vi "Dashboard Main.vi"() -> ()   [LabVIEW 2018]
uses:
  <vilib>/Utility/miscctls.llb/LVRowAndColumnTypeDef.ctl
  <vilib>/event_ctls.llb/eventvkey.ctl
  <vilib>/Rock Robotics/Network Tables/NT Read Numeric Array.vi
  <vilib>/Rock Robotics/WPI/Dashboard/WPI_DashboardLogging Global.vi
panel:
  in  "Camera Settings Right":T1={"Frame Rate"=30, "Compression"=30, "Size"=1, "DB Camera Config"=FALSE} {"Frame Rate" scale=1.0..30.0; "Compression" scale=100.0..-1.0; "Size" items=["640x480", "320x240", "160x120"]}
  in  "Camera Name Right":string(combo)="No Camera Selection"
  out "Camera Perf":string
  in  "Camera Settings":T1={"Frame Rate"=30, "Compression"=30, "Size"=1, "DB Camera Config"=FALSE} {"Frame Rate" scale=1.0..30.0; "Compression" scale=100.0..-1.0; "Size" items=["640x480", "320x240", "160x120"]}
  in  "TCP":refnum<k5>
  in  "Rec Mode":enum32{"Stop", "Record", "Playback"}(radio)
  out "Robot IP":string
  out "Image Message":string="Timeout in Camera Communications"
  in  "Dashboard Tab":T2(tab)=enum."Custom"
  in  "Select Auto":string(combo)="Select Autonomous ..."
  out "NT Connection":bool
  out "MotorChart R":cluster{"Numeric":dbl, "Numeric":dbl}(graph)
  out "MotorChart L":cluster{"Numeric":dbl, "Numeric":dbl}(graph)
  out "MotorSliders R":cluster{"MotorSlide1":dbl, "MotorSlide2":dbl} {"MotorSlide2" scale=-1.0..1.0 scale format="%#_2e"; "MotorSlide1" scale=-1.0..1.0 scale format="%#_2e"}
  out "MotorSliders L":cluster{"MotorSlide1":dbl, "MotorSlide2":dbl} {"MotorSlide2" scale=-1.0..1.0 scale format="%#_2e"; "MotorSlide1" scale=-1.0..1.0 scale format="%#_2e"}
  out "Gyro":dbl(knob) scale=0.0..360.0
  out "JS1 Z":dbl(slide) scale=-1.0..1.0 scale format="%#_2e"
  out "JS1 Graph":cluster{"X":dbl, "Y":dbl}[](graph)
  out "JS1 Buttons":T3
  out "JS2 Z":dbl(slide) scale=-1.0..1.0 scale format="%#_2e"
  out "JS2 Graph":cluster{"X":dbl, "Y":dbl}[](graph)
  out "JS2 Buttons":T3
  out "Mode":T4(ring)=enum."Auto Disabled"
  out "Right Camera Perf":cluster{"Bandwidth (Mbps)":dbl, "FPS":dbl}
  out "Camera Image Right":T5(plugin-control)
  in  "DB/String 9":string
  in  "DB/String 8":string
  in  "DB/String 7":string
  in  "DB/String 6":string
  in  "DB/String 5":string
  in  "DB/String 4":string
  in  "DB/String 3":string
  in  "DB/String 2":string
  in  "DB/String 1":string
  in  "DB/String 0":string
  in  "DB/Slider 0":dbl(slide) scale=0.0..5.0
  in  "DB/Slider 1":dbl(slide) scale=0.0..5.0
  in  "DB/Slider 2":dbl(slide) scale=0.0..5.0
  in  "DB/Slider 3":dbl(slide) scale=0.0..5.0
  out "DB/LED 3":bool
  out "DB/LED 2":bool
  out "DB/LED 1":bool
  out "DB/LED 0":bool
  in  "DB/Button 3":bool
  in  "DB/Button 2":bool
  in  "DB/Button 1":bool
  in  "DB/Button 0":bool caption="New Name"
  in  "Drift":dbl min=-5.0 max=5.0 step=0.1 format="%#_2g"
  in  "Rabbit":dbl=10.0 min=7.0 max=10.0 step=0.5
  in  "Speed":dbl=7.500000000000009 min=6.0 max=10.0 step=0.1 format="%#_2g"
  in  "Turtle":dbl=6.5 min=5.0 max=10.0 step=0.5 format="%#.1g"
  in  "Lift Speed":dbl=7.5 min=1.0 max=10.0 step=0.1
  in  "Tilt Speed":dbl=7.5 min=1.0 max=10.0 step=0.1
  in  "Kick Delay":dbl=0.05 min=0.05 max=1.0 step=0.05
  in  "Test Slider":dbl(slide) scale=0.0..100.0 scale format="%#_3g"
  in  "On/Off":bool caption="Solenoid"
  in  "Test Name":u16(ring) items=["Select the test to run..."]
  in  "Test Tree":string(tree)
  in  "Motor":cluster{"Value":dbl, "Enable":bool} {"Value" scale=-1.0..1.0 scale format="%#_3g"}
  out "Progress":T6 {"Test Progress" scale=0.0..100.0}
  in  "Rev/Fwd":cluster{"Forward":bool, "Reverse":bool}
  in  "Test Ring":u16(ring) items=["Monochrome", "Color"]
  out "Cmd Status":string
  in  "Execute Command":bool
  in  "Command Params":string[][](table)
  in  "Command Selection":i32(listbox)
  in  "CheckList":i32(listbox)
  out "Tree":string(tree)
  out "Camera Image":T5(plugin-control)
  out "Background":bool
  in  "Camera Name":string(combo)="No Camera Selection"
  # "HW"
  # "HW"
  # "Joysticks"
  # "Drive Motors"
  # "Front"
  # "Right"
  # "Left"
  # "Back"
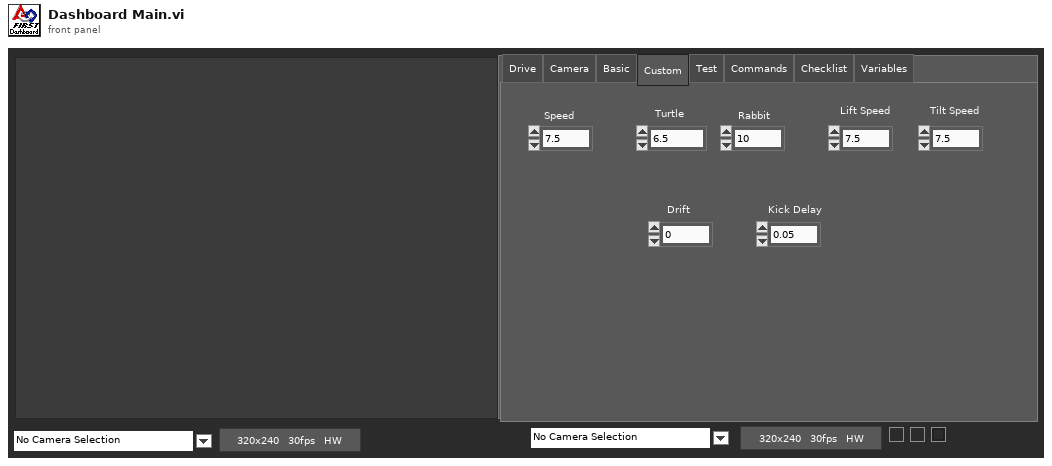
[diagram p1: front panel]
types:
  T1 = cluster{"Frame Rate":i32, "Compression":i32, "Size":u16, "DB Camera Config":bool}
  T2 = enum32{"Drive", "Camera", "Basic", "Custom", "Test", "Commands", "Checklist", "Variables"}
  T3 = cluster{bool, bool, bool, bool, bool, bool, bool, bool, bool, bool, bool, bool}
  T4 = enum8{"Tele-Op Disabled", "Tele-Op Enabled", "Auto Disabled", "Auto Enabled", "Test Disabled", "Test Enabled", "Disconnected", "No Code", "E-Stop"}
  T5 = typedef "IMAQ Image.ctl" = refnum<image>
  T6 = cluster{"Test Progress":u8, "Test Progress Text":string}
  T7 = cluster{"Save Path":path, "Interval (s)":dbl, "Keep":i32}
  T8 = typedef "Image Type" = u32
  T9 = cluster{"IDs":cluster{"RPC field ID":u16, "Unique ID":u16}, "String":string}
  T10 = cluster{"Error Strings":string, "Disable Counts":cluster{u16, u16}, "Rail Faults":cluster{u16, u16, u16}, "Robot IP":string, "DB Mode":u8, "Event Info":cluster{"Name":string, "Type":u8, "Number":u16, "Replay":u8}}
  T11 = cluster{"Storage":cluster{"Disk Free":u64, "RAM Block":u32, "RAM free":u32}, "CPU Utilization":cluster{"CPU % ISR":sgl, "CPU % Time Crit":sgl, "CPU % Timed Str":sgl, "CPU % High":sgl, "CPU % Above":sgl, "CPU % Normal":sgl, "CPU % Low":sgl}, "CAN":cluster{"% Bus Utilization":sgl, "Bus Off Cnt":u32, "TX_FIFO Full Cnt":u32, "Receive Error Cnt":u8, "Transmit Error Cnt":u8}, "HID":cluster{"HID Outputs":u32, "Rumble Low":u16, "Rumble High":u16}[]}
  T12 = cluster{"Status bits":cluster{"Test Mode":bool, "Autonomous":bool, "Enabled":bool, "Code Start":bool, "Brownout":bool, "Reserved 2":bool, "Reserved 3":bool, "E-Stop":bool}, "Code Trace":cluster{"Disabled":bool, "TeleOp":bool, "Auto":bool, "Test":bool}, "Controller Type":enum16{"unknown", "cRIO", "roboRio"}, "Code?":enum16{"unknown", "noCode", "code"}, "Battery V":dbl}
  T13 = cluster{"Control Bits":cluster{"TestMode":bool, "Autonomous":bool, "Enabled":bool, "FMS Present":bool, bool, bool, bool, "E-Stop":bool}, "Team Station ":u8, "Countdown":sgl, "Joystick Values":cluster{"Axes":dbl[], "Buttons":bool[], "POVs":i16[]}[]}
  T14 = cluster{"Axes":dbl[], "Buttons":bool[], "POVs":i16[]}[]
  T15 = cluster{"Axes":dbl[], "Buttons":bool[], "POVs":i16[]}
  T16 = cluster{"Buttons[0]":bool, "Buttons[1]":bool, "Buttons[2]":bool, "Buttons[3]":bool, "Buttons[4]":bool, "Buttons[5]":bool, "Buttons[6]":bool, "Buttons[7]":bool, "Buttons[8]":bool, "Buttons[9]":bool, "Buttons[10]":bool, "Buttons[11]":bool}
  T17 = cluster{"Camera Image":refnum<vi>, "Dashboard Tab":refnum<vi>, "Background":refnum<vi>, "Rec Mode":refnum<vi>, "Test Slider":refnum<vi>, "On/Off ":refnum<vi>, "Test Ring":refnum<vi>, "Rev/Fwd":refnum<vi>, "Test Name":refnum<vi>, "Motor":refnum<vi>, "Progress":refnum<vi>, "CheckList":refnum<vi>, "Tree":refnum<vi>, "Test Tree":refnum<vi>, "Command Params":refnum<vi>, "Command Selection":refnum<vi>, "Execute Command":refnum<vi>, "Cmd Status":refnum<vi>, "Camera Settings":refnum<vi>, "Camera Name":refnum<vi>, "Camera Perf":refnum<vi>, "Camera Settings Right":refnum<vi>, "Camera Name Right":refnum<vi>, "Camera Image Right":refnum<vi>}
  T18 = cluster{"Global Rectangle":i32[], "Contours":cluster{"Contour Type":u32, "ROI Type":u32, "Points":i32[]}[]}
  T19 = cluster{"Camera Name Right":string, string, "Saved DB Images Info":cluster{"Save Path":path, "Interval (s)":dbl, "Keep":i32}}
  T20 = cluster{"Camera Name":string, string, "Saved DB Images Info":cluster{"Save Path":path, "Interval (s)":dbl, "Keep":i32}}
  T21 = cluster{"Operation":enum16{"Update", "Clear"}, "Color Box":u32}[]
  T22 = typedef "eventvkey.ctl" = enum16{"ASCII", "Enter", "Return", "Shift", "Ctrl", "Alt", "Cmd", "Opt", "Caps", "NumLock", "Clear", "Break", "Up", "Down", "Left", "Right", "Insert", "Delete", "Home", "End", "PageUp", "PageDown", "Escape", "Help", "Pause", "ScrollLock", "F1", "F2", "F3", "F4", "F5", "F6", "F7", "F8", "F9", "F10", "F11", "F12", "F13", "F14", "F15", "F16", "F17", "F18", "F19", "F20", "F21", "F22", "F23", "F24", "Play", "VolumeUp", "VolumeDown", "Mute", "Two Byte Char"}
  T23 = cluster{"Image Size":bool, "Image Type":bool, "Pixel Value":bool, "ROI Information":bool, "Zoom Factor":bool}
  T24 = cluster{"Operation":enum16{"Update", "Clear"}, "Color Box":u32}
  T25 = typedef "LVRowAndColumnTypeDef.ctl" = cluster{"Row":i32, "Column":i32}
  T26 = cluster{"Shift":bool, "Ctrl":bool, "Alt":bool, "Cmd":bool, "Opt":bool}
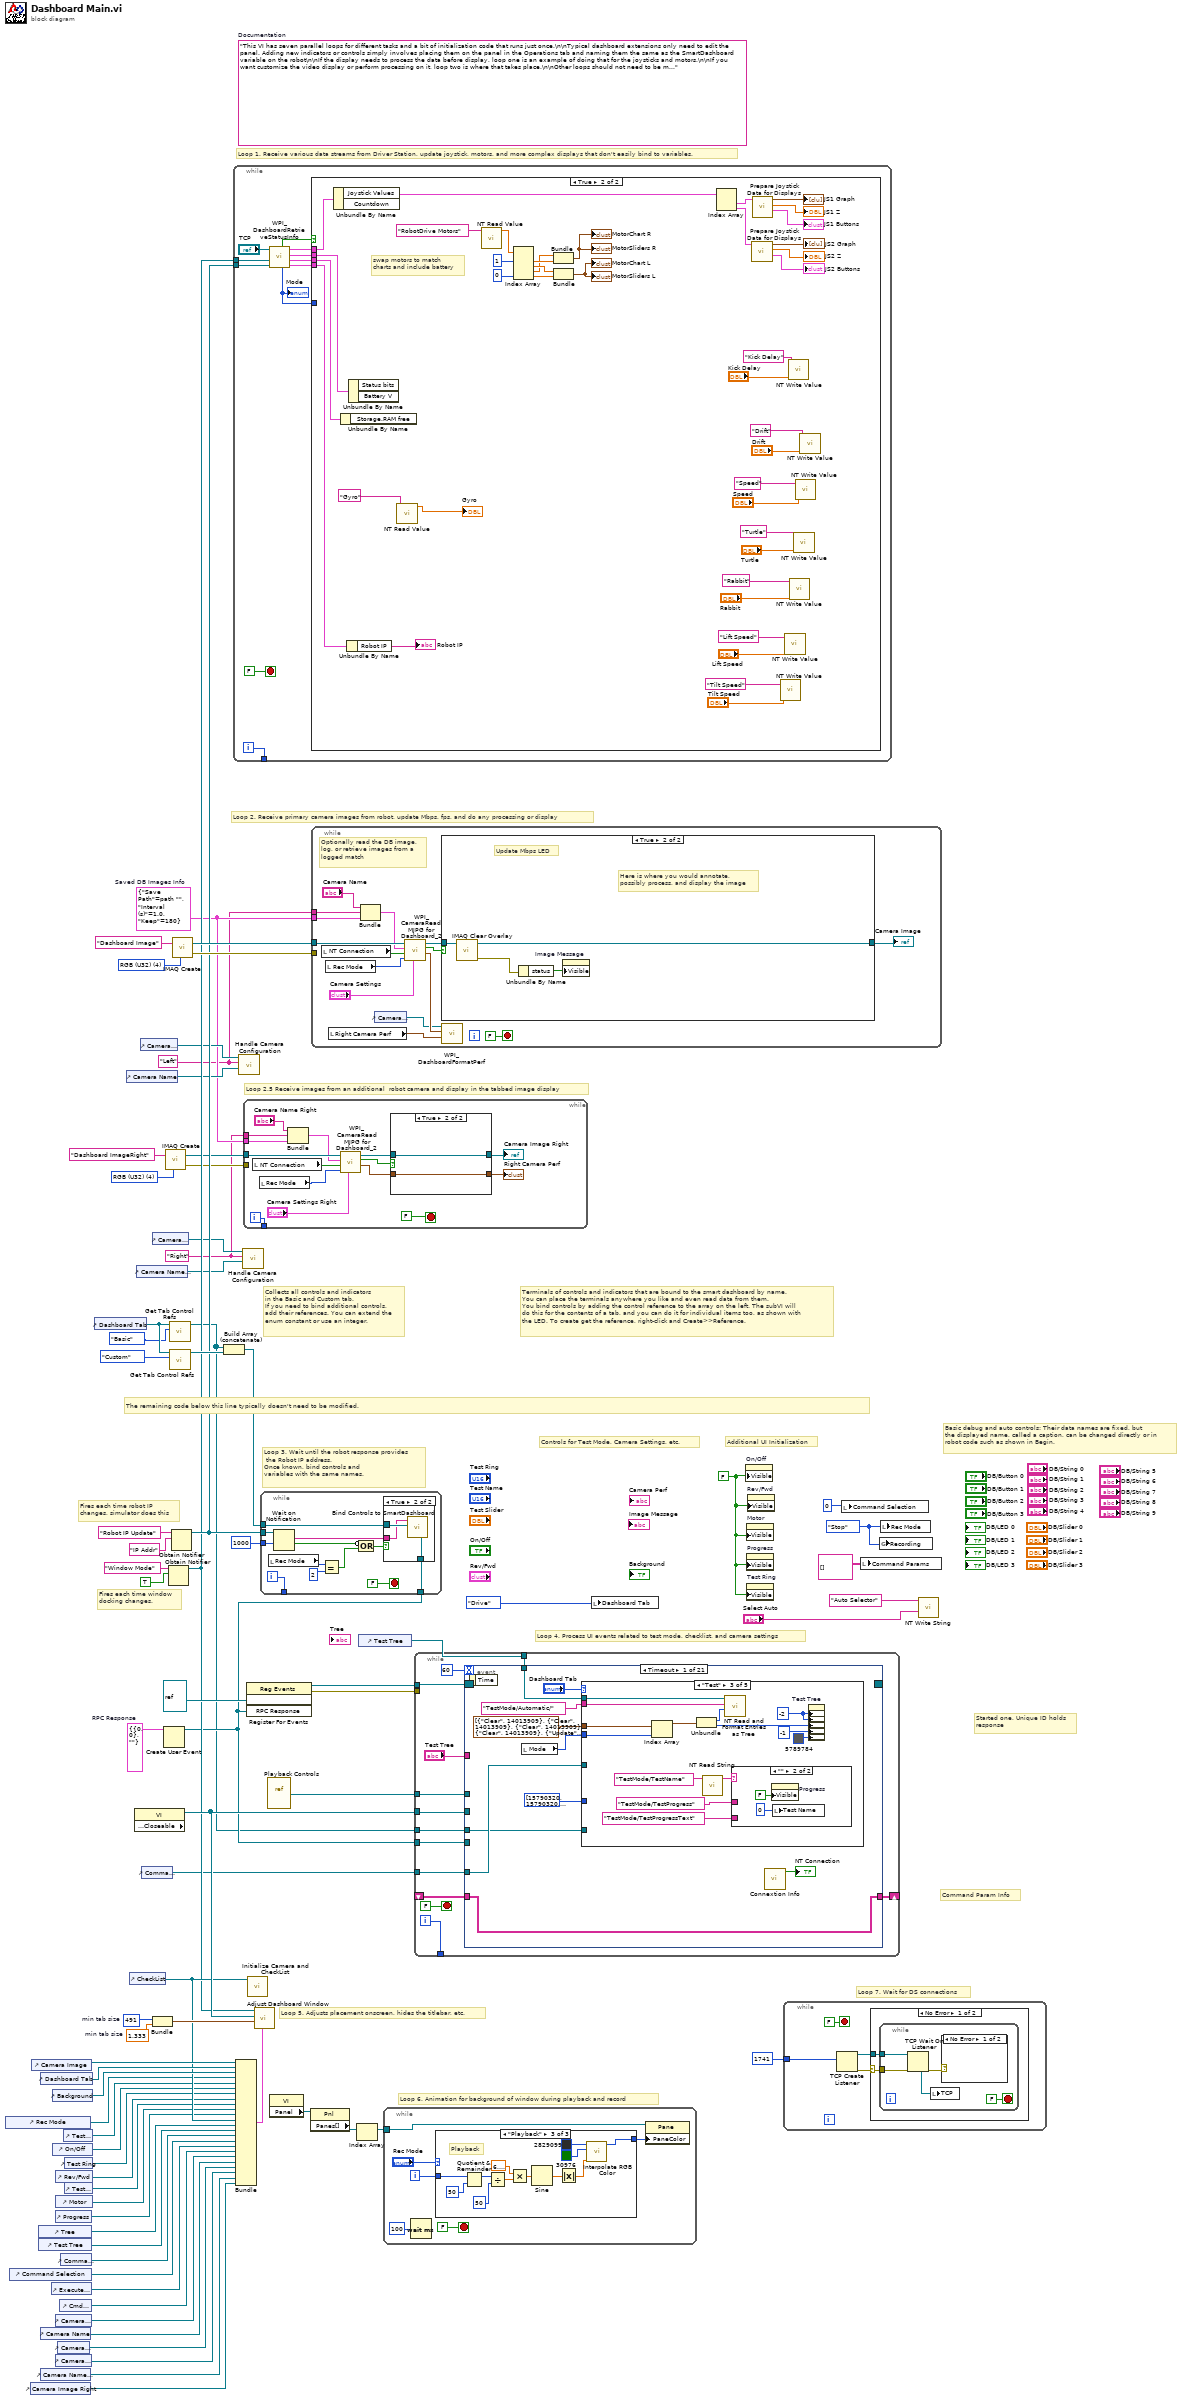
[diagram p0: block diagram]
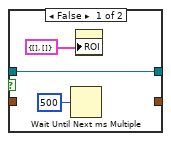
[diagram p2: hidden frame]
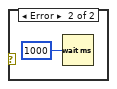
[diagram p3: hidden frame]
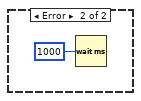
[diagram p4: hidden frame]
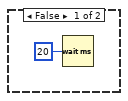
[diagram p5: hidden frame]
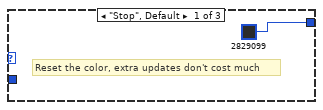
[diagram p6: hidden frame]
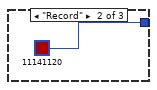
[diagram p7: hidden frame]
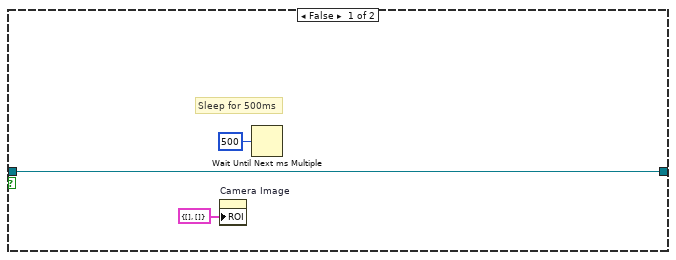
[diagram p9: hidden frame]
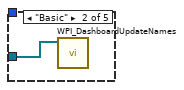
[diagram p11: hidden frame]
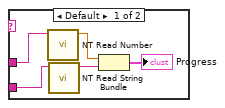
[diagram p12: hidden frame]
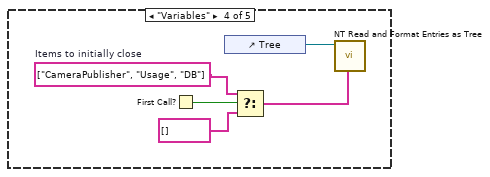
[diagram p13: hidden frame]
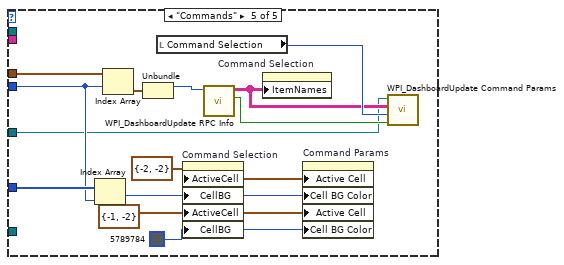
[diagram p14: hidden frame]
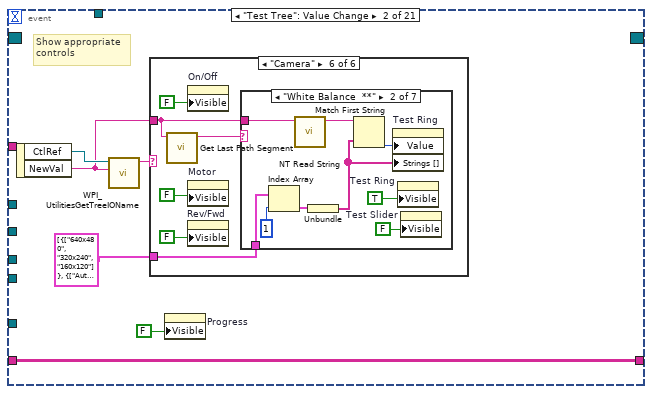
[diagram p15: hidden frame]
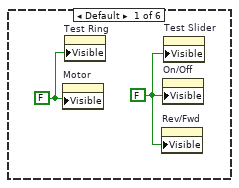
[diagram p16: hidden frame]
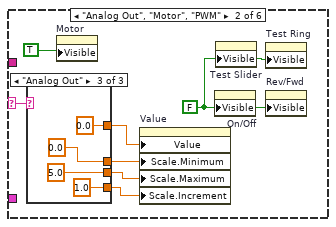
[diagram p17: hidden frame]
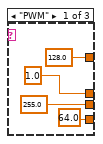
[diagram p18: hidden frame]
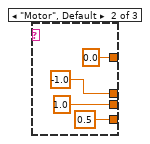
[diagram p19: hidden frame]
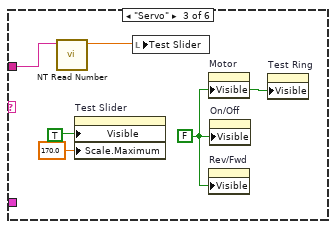
[diagram p20: hidden frame]
diagram:
  w3 = T7 {"Save Path"=path "", "Interval (s)"=1.0, "Keep"=180}  # Saved DB Images Info
  w2 = "Right"
  w1 = "Left"
  w13 = T8 4 items=["Grayscale (U8)", "Grayscale (I16)", "Grayscale (SGL)", "Complex (CSG)", "RGB (U32)", "HSL (U32)", "RGB (U64)"] ("Image Type")
  w29 = T9 {"IDs"={"RPC field ID"=0, "Unique ID"=0}, "String"=""}  # RPC Response
  w52 = 491  # min tab size
  w51 = 1.333  # min tab size
  w59 = enum32{"Stop", "Record", "Playback"}."Stop" ("Rec Mode")
  w36 = FALSE ("Visible")
  (unwired) "This VI has seven parallel loops for different tasks and a bit of initialization code that runs just once.\n\nTypical dashboard extensions only need to edit the panel. Adding new indicators or controls simply involves placing them on the panel in the Operations tab and naming them the same as the SmartDashboard variable on the robot\n\nIf the display needs to process the data before display, loop one is an example of doing that for the joysticks and motors.\n\nIf you want customize the video display or perform processing on it, loop two is where that takes place.\n\nOther loops should not need to be modified. They are pretty standard, and document the task they perform."  # Documentation
  w76 = T8 4 items=["Grayscale (U8)", "Grayscale (I16)", "Grayscale (SGL)", "Complex (CSG)", "RGB (U32)", "HSL (U32)", "RGB (U64)"] ("Image Type")
  # "Loop 2.5 Receive images from an additional  robot camera and display in the tabbed image display"
  # "Command Param Info"
  # "Started one, Unique ID holds\nresponse"
  # "Loop 7. Wait for DS connections"
  # "Basic debug and auto controls: Their data names are fixed, but\nthe displayed name, called a caption, can be changed directly or in\nrobot code such as shown in Begin."
  # "Controls for Test Mode, Camera Settings, etc."
  # "Additional UI Initialization"
  # "Loop 6. Animation for background of window during playback and record"
  # "Fires each time robot IP\nchanges, simulator does this"
  # "Fires each time window\ndocking changes."
  # "Collects all controls and indicators\nin the Basic and Custom tab.\nIf you need to bind additional controls,\nadd their references. You can extend the\nenum constant or use an integer."
  # "The remaining code below this line typically doesn't need to be modified."
  # "Loop 4. Process UI events related to test mode, checklist, and camera settings"
  # "Terminals of controls and indicators that are bound to the smart dashboard by name.\nYou can place the terminals anywhere you like and even read data from them.\nYou bind controls by adding the control reference to the array on the left. The subVI will\ndo this for the contents of a tab, and you can do it for individual items too, as shown with\nthe LED. To create get the reference, right-click and Create>>Reference."
  # "Loop 3. Wait until the robot response provides\n the Robot IP address.\nOnce known, bind controls and\nvariables with the same names."
  # "Loop 5. Adjusts placement onscreen, hides the titlebar, etc."
  # "Loop 1. Receive various data streams from Driver Station, update joystick, motors, and more complex displays that don't easily bind to variables."
  # "Loop 2. Receive primary camera images from robot, update Mbps, fps, and do any processing or display"
  n1 = control-ref of="Rec Mode"() -> (w42:refnum<vi>)
  n2 = control-ref of="Command Selection"() -> (w28:refnum<vi>)
  n3 = control-ref of="Camera Image Right"() -> (w6:refnum<vi>)
  n4 = control-ref of="Camera Image"() -> (w54:refnum<vi>)
  n5 = control-ref of="Tree"() -> (w46:refnum<vi>)
  n6 = control-ref of="Test Tree"() -> (w45:refnum<vi>)
  n7 = control-ref of="Dashboard Tab"() -> (w53:refnum<vi>)
  n8 = control-ref of="Camera Name"() -> (w19:refnum<vi>)
  n9 = control-ref of="Camera Name Right"() -> (w7:refnum<vi>)
  n10 = control-ref of="Execute Command"() -> (w30:refnum<vi>)
  n11 = control-ref of="Background"() -> (w49:refnum<vi>)
  n12 = control-ref of="On/Off"() -> (w40:refnum<vi>)
  n13 = control-ref of="Progress"() -> (w37:refnum<vi>)
  n14 = control-ref of="Camera Settings"() -> (w20:refnum<vi>)
  n15 = control-ref of="Camera Settings Right"() -> (w8:refnum<vi>)
  n16 = control-ref of="Rev/Fwd"() -> (w38:refnum<vi>)
  n17 = control-ref of="Motor"() -> (w43:refnum<vi>)
  n18 = control-ref of="Camera Perf"() -> (w18:refnum<vi>)
  n19 = control-ref of="Cmd Status"() -> (w24:refnum<vi>)
  n20 = control-ref of="Command Params"() -> (w31:refnum<vi>)
  n21 = control-ref of="Test Slider"() -> (w41:refnum<vi>)
  n22 = control-ref of="Test Ring"() -> (w39:refnum<vi>)
  n23 = control-ref of="Test Name"() -> (w44:refnum<vi>)
  n24 = control-ref of="Dashboard Tab"() -> (w57:refnum<vi>)
  n25 = control-ref of="Camera Name"() -> (w21:refnum<vi>)
  n26 = control-ref of="CheckList"() -> (w47:refnum<vi>)
  n27 = property class="VI" props=["Front Panel.Closeable"]() -> (reference out=w58:refnum<vi>)  [unwired: 2 in, 2 out]
  n28 = control-ref of="Camera Name Right"() -> (w9:refnum<vi>)
  n29 = control-ref of="Camera Settings"() -> (w22:refnum<vi>)
  n30 = control-ref of="Command Params"() -> (w23:refnum<vi>)
  n31 = control-ref of="Camera Settings Right"() -> (w10:refnum<vi>)
  n32 = Bundle("min tab size"=w52, "min tab size"=w51) -> (w50:cluster{"min tab size":i32, "min tab size":dbl})  [unwired: 1 in]
  n33 = Create User Event(user event datatype=w29) -> (user event=w25:refnum<user-event>)  [unwired: 1 in, 1 out]
  n34 = call "IMAQ Create"("Image Name"="Dashboard ImageRight", "Image Type"=w13) -> ("New Image"=w12:T5, "error out"=w11:errorcluster)  [unwired: 2 in, 1 out]
  n35 = Obtain Notifier(name (unnamed)="Window Mode", notification data type=TRUE) -> (notifier out=w34:refnum<notifier>)  [unwired: 2 in, 2 out]
  n36 = call <vilib>:"Get Tab Control Refs.vi"("Page Index"=T2."Basic" ("Dashboard Tab"), "TabControl in"=w57) -> ("ControlsOnPage"=w17:refnum<vi>[])  [unwired: 9 in]
  n37 = call <vilib>:"Get Tab Control Refs.vi"("Page Index"=T2."Custom" ("Dashboard Tab"), "TabControl in"=w57) -> ("ControlsOnPage"=w56:refnum<vi>[])  [unwired: 9 in]
  n38 = Obtain Notifier(name (unnamed)="Robot IP Update", notification data type="IP Addr" ("name (unnamed)")) -> (notifier out=w35:refnum<notifier>)  [unwired: 2 in, 2 out]
  n39 = call "IMAQ Create"("Image Name"="Dashboard Image", "Image Type"=w76) -> ("New Image"=w74:T5, "error out"=w73:errorcluster)  [unwired: 2 in, 1 out]
  n40 = Build Array (concatenate)(w17, w56) -> (w55:refnum<vi>[])
  n41 = while {
    tunnel: [w86] -> _
    tunnel: w35 -> [w80]
    tunnel: w34 -> [w77]
    i -> [w86]
    stop <- FALSE stop-if-true
    n42 = call <vilib>:"WPI_DashboardRetrieveStatusInfo.vi"("Binding Refnum"=w80, "Window Mode Notifier"=w77, "TCP Cnx"="TCP") -> ("Power and Errors"=w81:T10, "Robot Metrics"=w84:T11, "Status Info"=w85:T12, "Control Info"=w82:T13, "Robot Mode"=w79:T4, "Process?"=w83:bool)  [unwired: 3 in]
    "Mode" <- w79
    n43 = case shown="True" w83 {
      tunnel: w85 -> [_ w128]
      tunnel: w84 -> [_ w127]
      tunnel: w82 -> [_ w126]
      tunnel: w81 -> [_ w125]
      tunnel: w79 -> [_ _]
      frame False {
        n44 = Wait (ms)(milliseconds to wait=u32 20) -> ()  [unwired: 1 out]
      }
      frame True {
        # "swap motors to match\ncharts and include battery"
        n45 = Unbundle By Name(w126) -> ("Joystick Values"=w116:T14)  [unwired: 1 out]
        n46 = Unbundle By Name(w127) -> ()  [unwired: 1 out]
        n47 = Unbundle By Name(w125) -> ("Robot IP"=→"Robot IP":string)
        n48 = Unbundle By Name(w128) -> ()  [unwired: 2 out]
        n49 = call-poly <vilib>:"NT Read Value.vi"("Name"="Gyro") -> ("Numeric"=→"Gyro":dbl)  [unwired: 9 in, 1 out]
        n50 = call-poly <vilib>:"NT Read Value.vi"("Name"="RobotDrive Motors") -> ("Numeric Array"=w106:dbl[])  [unwired: 9 in, 1 out]
        n51 = Index Array(array=w106, index #1=1, index #4=0) -> (element #1=w120:dbl, element #2=w121:dbl, element #3=w119:dbl, element #4=w124:dbl)  [unwired: 2 in]
        n52 = Bundle("Numeric"=w119, "Numeric"=w120) -> (→"MotorChart R" →"MotorSliders R":cluster{"Numeric":dbl, "Numeric":dbl})  [unwired: 1 in]
        n53 = Bundle("Numeric"=w121, "Numeric"=w124) -> (→"MotorChart L" →"MotorSliders L":cluster{"Numeric":dbl, "Numeric":dbl})  [unwired: 1 in]
        n54 = Index Array(array=w116) -> (element #1=w115:T15, element #2=w111:T15)  [unwired: 2 in]
        n55 = call "Prepare Joystick Data for Displays.vi"("Joystick Values"=w111) -> ("Buttons"=→"JS2 Buttons":T16, "Z Axis"=→"JS2 Z":dbl, "Cartesian Data"=→"JS2 Graph":cluster{"X axis":dbl, "X axis":dbl}[])  [unwired: 8 in]
        n56 = call "Prepare Joystick Data for Displays.vi"("Joystick Values"=w115) -> ("Buttons"=→"JS1 Buttons":T16, "Z Axis"=→"JS1 Z":dbl, "Cartesian Data"=→"JS1 Graph":cluster{"X axis":dbl, "X axis":dbl}[])  [unwired: 8 in]
        n57 = call-poly <vilib>:"NT Write Value.vi"("Numeric"="Tilt Speed", "Name"="Tilt Speed") -> ()  [unwired: 9 in, 1 out]
        n58 = call-poly <vilib>:"NT Write Value.vi"("Numeric"="Lift Speed", "Name"="Lift Speed") -> ()  [unwired: 9 in, 1 out]
        n59 = call-poly <vilib>:"NT Write Value.vi"("Numeric"="Kick Delay", "Name"="Kick Delay") -> ()  [unwired: 9 in, 1 out]
        n60 = call-poly <vilib>:"NT Write Value.vi"("Numeric"="Rabbit", "Name"="Rabbit") -> ()  [unwired: 9 in, 1 out]
        n61 = call-poly <vilib>:"NT Write Value.vi"("Numeric"="Turtle", "Name"="Turtle") -> ()  [unwired: 9 in, 1 out]
        n62 = call-poly <vilib>:"NT Write Value.vi"("Numeric"="Speed", "Name"="Speed") -> ()  [unwired: 9 in, 1 out]
        n63 = call-poly <vilib>:"NT Write Value.vi"("Numeric"="Drift", "Name"="Drift") -> ()  [unwired: 9 in, 1 out]
      }
    }
  }
  n64 = Bundle("Camera Image"=w54, "Dashboard Tab"=w53, "Background"=w49, "Rec Mode"=w42, "Test Slider"=w41, "On/Off"=w40, "Test Ring"=w39, "Rev/Fwd"=w38, "Test Name"=w44, "Motor"=w43, "Progress"=w37, "CheckList"=w47, "Tree"=w46, "Test Tree"=w45, "Command Params"=w31, "Command Selection"=w28, "Execute Command"=w30, "Cmd Status"=w24, "Camera Settings"=w20, "Camera Name"=w19, "Camera Perf"=w18, "Camera Settings Right"=w8, "Camera Name Right"=w7, "Camera Image Right"=w6) -> (w48:T17)  [unwired: 1 in]
  n65 = call "Handle Camera Configuration.vi"("CameraNameRef"=w21, "Display Name"=w1, "ClusterRef"=w22) -> ()  [unwired: 9 in]
  n66 = call "Handle Camera Configuration.vi"("CameraNameRef"=w9, "Display Name"=w2, "ClusterRef"=w10) -> ()  [unwired: 9 in]
  n67 = while {
    tunnel: w12 -> [w143]
    tunnel: w11 -> [_]
    tunnel: [w138] -> _
    tunnel: w3 -> [w134]
    tunnel: w2 -> [w131]
    i -> [w138]
    stop <- FALSE stop-if-true
    n68 = local read "NT Connection"() -> (w135:bool)
    n69 = local read "Rec Mode"() -> (w142:enum32{"Stop", "Record", "Playback"})
    n70 = Bundle("Camera Name Right"="Camera Name Right", w131, "Saved DB Images Info"=w134) -> (w133:T19)  [unwired: 1 in]
    n71 = call <vilib>:"WPI_CameraRead MJPG for Dashboard_2.vi"("Camera Settings"="Camera Settings Right", "Rec Mode"=w142, "NT Connection"=w135, "Capture Info"=w133, "Image in"=w143) -> ("perf info"=w129:cluster{"Bandwidth (Mbps)":dbl, "fps":dbl}, "Active"=w137:bool, "Image\\ out"=w140:T5)  [unwired: 4 in]
    n72 = case shown="True" w137 {
      tunnel: w140 -> [w145 w148]
      tunnel: [w145 w148] -> w136
      tunnel: [_ w147] -> w130
      tunnel: w129 -> [_ w147]
      frame False {
        n73 = Wait Until Next ms Multiple(millisecond multiple=u32 500) -> ()  [unwired: 1 out]
        n74 = property on="Camera Image Right" class="ImageControl"("ROI"=T18 {"Global Rectangle"=[], "Contours"=[]}) -> ()  [unwired: 2 in, 2 out]
      }
      frame True {
      }
    }
    "Camera Image Right" <- w136
    "Right Camera Perf" <- w130
  }
  n75 = register-events(refnum<vi> refnum, w25) -> (reference out=w63:refnum<event-registration>, error out=w62:errorcluster)  [unwired: 2 in]
  n76 = call "Initialize Camera and CheckList.vi"("ListBox in"=w47) -> ()  [unwired: 11 in]
  n77 = call "Adjust Dashboard Window.vi"("Sizing Refnums"=w48, "Size Constraints"=w50, "VI"=w58, "WIn Mode"=w34) -> ()  [unwired: 8 in]
  n78 = while {
    tunnel: w55 -> [w160]
    tunnel: w35 -> [w158]
    tunnel: [w156] -> _
    tunnel: u32 1000 ("milliseconds to wait") -> [w155]
    tunnel: w25 -> [w149]
    i -> [w156]
    stop <- FALSE stop-if-true
    n79 = local read "Rec Mode"() -> (w151:enum32{"Stop", "Record", "Playback"})
    n80 = Wait on Notification(notifier=w158, timeout in ms (-1)=w155) -> (notification=w157:string, timed out?=w153:bool)  [unwired: 2 in, 2 out]
    n81 = Equal?(x=w151, y=u16 2 ("Rec Mode")) -> (x = y?=w152:bool)
    n82 = Compound Arithmetic op=OR(invert w153, w152) -> (w154:bool)
    n83 = case shown="True" w154 {
      tunnel: w160 -> [_ w163]
      tunnel: w157 -> [_ w162]
      tunnel: w149 -> [_ w161]
      frame False {
      }
      frame True {
        n84 = call <vilib>:"Bind Controls to SmartDashboard.vi"("RPC ref"=w161, "Bound Control Refs"=w163, "Server IP Address"=w162) -> ()  [unwired: 9 in]
      }
    }
  }
  n85 = vi-ref "Playback Controls.vi"() -> (w64:refnum<vi>)
  n86 = property class="VI"() -> ("Panel"=w66:refnum<vi>)  [unwired: 2 in, 2 out]
  n87 = property class="Pnl"(reference=w66) -> ("Panes[]"=w67:refnum<vi>[])  [unwired: 1 in, 2 out]
  n88 = while {
    tunnel: w74 -> [w177]
    tunnel: w73 -> [_]
    tunnel: w3 -> [w170]
    tunnel: w1 -> [w167]
    stop <- FALSE stop-if-true
    # "Optionally read the DB image,\nlog, or retrieve images from a\nlogged match"
    n89 = local read "NT Connection"() -> (w171:bool)
    n90 = local read "Rec Mode"() -> (w174:enum32{"Stop", "Record", "Playback"})
    n91 = local read "Right Camera Perf"() -> (w165:cluster{"Bandwidth (Mbps)":dbl, "FPS":dbl})
    n92 = Bundle("Camera Name"="Camera Name", w167, "Saved DB Images Info"=w170) -> (w169:T20)  [unwired: 1 in]
    n93 = control-ref of="Camera Perf"() -> (w164:refnum<vi>)
    n94 = call <vilib>:"WPI_CameraRead MJPG for Dashboard_2.vi"("Camera Settings"="Camera Settings", "Rec Mode"=w174, "NT Connection"=w171, "Capture Info"=w169, "Image in"=w177) -> ("perf info"=w166:cluster{"Bandwidth (Mbps)":dbl, "fps":dbl}, "Active"=w175:bool, "Image\\ out"=w176:T5)  [unwired: 4 in]
    n95 = case shown="True" w175 {
      tunnel: w176 -> [w180 w183]
      tunnel: [w180 w182] -> w172
      frame False {
        # "Sleep for 500ms"
        n96 = property on="Camera Image" class="ImageControl"("ROI"=T18 {"Global Rectangle"=[], "Contours"=[]}) -> ()  [unwired: 2 in, 2 out]
        n97 = Wait Until Next ms Multiple(millisecond multiple=u32 500) -> ()  [unwired: 1 out]
      }
      frame True {
        # "Here is where you would annotate,\npossibly process, and display the image"
        # "Update Mbps LED"
        n98 = call "IMAQ Clear Overlay"("Image"=w183) -> ("error out"=w184:errorcluster, "Image Out"=w182:T5)  [unwired: 2 in, 7 out]
        n99 = Unbundle By Name(w184) -> ("status"=w185:bool)
        n100 = property on="Image Message" class="Str"("Visible"=w185) -> ()  [unwired: 2 in, 2 out]
      }
    }
    "Camera Image" <- w172
    n101 = call <vilib>:"WPI_DashboardFormatPerf.vi"("Right Camera Perf"=w165, "Performance"=w166, "String in"=w164) -> ()  [unwired: 9 in]
  }
  n102 = Index Array(array=w67) -> (element=w65:refnum<vi>)  [unwired: 1 in]
  n103 = control-ref of="Test Tree"() -> (w68:refnum<vi>)
  n104 = while {
    tunnel: w65 -> [w187]
    i -> [w190]
    stop <- FALSE stop-if-true
    n105 = Wait (ms)(milliseconds to wait=u32 100) -> ()  [unwired: 1 out]
    n106 = case shown="\"Playback\"" "Rec Mode" {
      tunnel: w190 -> [_ _ w205]
      tunnel: [u32 2829099 ("Base Color") u32 11141120 ("Target Color") w194] -> w186
      frame "Stop", Default {
        # "Reset the color, extra updates don't cost much"
      }
      frame "Record" {
      }
      frame "Playback" {
        # "Playback"
        n107 = Quotient & Remainder(x=w205, y=u32 50 ("milliseconds to wait")) -> (x-y*floor(x/y)=w201:u32)  [unwired: 1 out]
        n108 = Divide(x=w201, y=u32 50 ("milliseconds to wait")) -> (x/y=w198:dbl)
        n109 = Multiply(x=6.283185307179586, y=w198) -> (x*y=w203:dbl)
        n110 = Sine(x=w203) -> (sin(x)=w202:dbl)
        n111 = Absolute Value(x=w202) -> (abs(x)=w195:dbl)
        n112 = call "Interpolate RGB Color.vi"("Proportion"=w195, "Target Color"=u32 30976, "Base Color"=u32 2829099) -> ("Result Color"=w194:u32)  [unwired: 8 in]
      }
    }
    n113 = property class="Pane"(reference=w187, "PaneColor"=w186) -> ()  [unwired: 1 in, 2 out]
  }
  n114 = while {
    tunnel: [w215] -> _
    tunnel: w68 -> [w214]
    tunnel: w64 -> [w213]
    tunnel: w63 -> [w212]
    tunnel: w62 -> [_]
    tunnel: w58 -> [w211]
    tunnel: w25 -> [w210]
    tunnel: w23 -> [w209]
    shift-right: [w208] -> _
    shift-left: _ -> [w207]
    tunnel: w17 -> [w206]
    i -> [w215]
    stop <- FALSE stop-if-true
    n115 = event shown="[0] Timeout" {
      selector: w212 -> [_ _ _ _ _ _ _ _ _ _ _ _ _ _ _ _ _ _ _ _ _]
      dyn-events: [_ _ _ _ _ _ _ _ _ _ _ _ _ _ _ _ w475 _ _ _ _] -> _
      timeout: u32 60 ("milliseconds to wait") -> [_ _ _ _ _ _ _ _ _ _ _ _ _ _ _ _ _ _ _ _ _]
      tunnel: w214 -> [w227 _ _ _ _ _ _ _ _ _ _ _ _ _ _ _ _ _ _ _ _]
      tunnel: "Test Tree" -> [_ _ _ _ _ _ _ _ _ _ _ w442 w450 w452 w456 w464 _ _ _ _ _]
      tunnel: w213 -> [_ _ _ _ _ _ _ _ _ _ _ _ _ _ _ _ w477 _ w495 _ _]
      tunnel: w211 -> [_ _ _ _ _ _ _ _ _ _ _ _ _ _ _ _ w473 _ _ _ _]
      tunnel: w210 -> [_ _ _ _ _ _ _ _ _ _ _ _ _ _ _ _ w471 _ _ _ _]
      tunnel: w209 -> [w222 _ _ _ _ _ w393 _ _ _ _ _ _ _ _ _ _ _ _ _ _]
      tunnel: [w221 w270 w372 w377 w386 w390 w391 w400 w410 w417 w429 w441 w448 w451 w455 w463 w470 w490 w492 w496 w509] -> w208
      tunnel: w207 -> [w221 w270 w372 w377 w386 w390 w391 _ _ w417 w429 w441 w448 w451 w455 w463 w470 w490 w492 w496 w509]
      tunnel: w206 -> [w219 _ _ _ _ _ _ _ _ _ _ _ _ _ _ _ _ _ _ _ _]
      event Timeout {
        n116 = event-data() -> ()  [unwired: 1 in, 1 out]
        n117 = local read "Mode"() -> (w224:T4)
        n118 = case shown="\"Test\"" "Dashboard Tab" {
          tunnel: w227 -> [_ _ w243 _ _]
          tunnel: "TestMode/Automatic/" ("Name Pattern") -> [_ _ w242 _ _]
          tunnel: T21 [{"Operation"=enum."Clear", "Color Box"=14013909}, {"Operation"=enum."Clear", "Color Box"=14013909}, {"Operation"=enum."Clear", "Color Box"=14013909}, {"Operation"=enum."Clear", "Color Box"=14013909}, {"Operation"=enum."Update", "Color Box"=14013909}, {"Operation"=enum."Update", "Color Box"=16777215}, {"Operation"=enum."Clear", "Color Box"=14013909}, {"Operation"=enum."Clear", "Color Box"=14013909}, {"Operation"=enum."Clear", "Color Box"=14013909}] -> [_ _ w235 _ w263]
          tunnel: w224 -> [_ _ w234 _ w262]
          tunnel: u32[] [15790320, 15790320, 15790320, 15790320, 16777215, 16777215, 15790320, 15790320, 15790320] -> [_ _ _ _ w268]
          tunnel: w222 -> [_ _ _ _ w256]
          tunnel: w219 -> [_ w229 _ _ _]
          frame "Custom", Default {
          }
          frame "Basic" {
            n119 = call <vilib>:"WPI_DashboardUpdateNames.vi"("Controls on Tab"=w229) -> ()  [unwired: 11 in]
          }
          frame "Test" {
            w241 = -2 ("Active Item:Row Number")
            n120 = Index Array(array=w235, index=w234) -> (element=w236:T24)
            n121 = Unbundle(w236) -> ("Operation"=w237:enum16{"Update", "Clear"}, "Color Box"=w238:u32)
            n122 = call <vilib>:"NT Read String.vi"("Name"="TestMode/TestName") -> ("String"=w232:string)  [unwired: 9 in, 1 out]
            n123 = call <vilib>:"NT Read and Format Entries as Tree.vi"("Operation"=w237, "Name Pattern"=w242, "Tree Refnum"=w243) -> ()  [unwired: 7 in, 2 out]
            n124 = case shown="\"\"" w232 {
              tunnel: "TestMode/TestProgress" ("Name") -> [w245 _]
              tunnel: "TestMode/TestProgressText" ("Name") -> [w244 _]
              frame Default {
                n125 = call <vilib>:"NT Read Number.vi"("Name"=w245) -> ("Numeric"=w246:dbl)  [unwired: 9 in, 1 out]
                n126 = call <vilib>:"NT Read String.vi"("Name"=w244) -> ("String"=w247:string)  [unwired: 9 in, 1 out]
                n127 = Bundle("Numeric"=w246, "String"=w247) -> (→"Progress":cluster{"Numeric":dbl, "String":string})  [unwired: 1 in]
              }
              frame "" {
                n128 = property on="Progress" class="Clust (strict)"("Visible"=FALSE) -> ()  [unwired: 2 in, 2 out]
                n129 = local write "Test Name"(u16 0) -> ()
              }
            }
            n130 = property on="Test Tree" class="Tree (strict)"("Active Item Row Number"=w241, "ActiveColNum"=w241, "CellBG"=w238, "Active Item Row Number"=-1 ("Active Item:Row Number"), "CellBG"=u32 5789784 ("Color Box")) -> ()  [unwired: 2 in, 2 out]
          }
          frame "Variables" {
            w253 = string[] ["CameraPublisher", "Usage", "DB"]  # Items to initially close
            n131 = First Call?() -> (First Call?: T/F=w254:bool)
            n132 = control-ref of="Tree"() -> (w255:refnum<vi>)
            n133 = Select(t=w253, s=w254, f=string[] []) -> (s? t:f=w251:string[])
            n134 = call <vilib>:"NT Read and Format Entries as Tree.vi"("Tags to  Close"=w251, "Tree Refnum"=w255) -> ()  [unwired: 8 in, 2 out]
          }
          frame "Commands" {
            w264 = u32 5789784 ("Color Box")
            w265 = T25 {"Row"=-1, "Column"=-2} ("Active Cell:Active Cell")
            w267 = T25 {"Row"=-2, "Column"=-2} ("Active Cell:Active Cell")
            n135 = Index Array(array=w268, index=w262) -> (element=w266:u32)
            n136 = Index Array(array=w263, index=w262) -> (element=w261:T24)
            n137 = Unbundle(w261) -> ("Operation"=w260:enum16{"Update", "Clear"})  [unwired: 1 out]
            n138 = local read "Command Selection"() -> (w259:i32)
            n139 = property on="Command Selection" class="MCListbox (strict)"("ActiveCell"=w267, "CellBG"=w266, "ActiveCell"=w265, "CellBG"=w264) -> ()  [unwired: 2 in, 2 out]
            n140 = call <vilib>:"WPI_DashboardUpdate RPC Info.vi"("Operation"=w260) -> ("update"=w258:bool, "commands"=w257:string[][])  [unwired: 9 in]
            n141 = property on="Command Selection" class="MCListbox (strict)"("ItemNames"=w257) -> ()  [unwired: 2 in, 2 out]
            n142 = property on="Command Params" class="Tbl (strict)"("Active Cell"=w267, "Cell BG Color"=w266, "Active Cell"=w265, "Cell BG Color"=w264) -> ()  [unwired: 2 in, 2 out]
            n143 = call <vilib>:"WPI_DashboardUpdate Command Params.vi"("Update"=w258, "NewVal"=w259, "Commands"=w257, "Param Tbl"=w256) -> ()  [unwired: 7 in, 1 out]
          }
        }
        n144 = call <vilib>:"Connextion Info.vi"() -> ("Connected"=→"NT Connection":bool)  [unwired: 10 in, 1 out]
      }
      event "Test Tree": Value Change {
        # "Show appropriate\ncontrols"
        n145 = event-data() -> ("CtlRef"=w273:refnum<vi>, "NewVal"=w271:string)  [unwired: 1 in]
        n146 = call <vilib>:"WPI_UtilitiesGetTreeIOName.vi"("NewVal"=w271, "TreeControl in"=w273) -> ("I/O Name"=w274:string)  [unwired: 9 in]
        n147 = case shown="\"Camera\"" w274 {
          selector: w274 -> [_ w281 _ w303 w312 _]
          tunnel: w271 -> [_ _ w300 w302 _ w319]
          tunnel: cluster{string[]}[] [{["640x480", "320x240", "160x120"]}, {["Auto", "Fixed indoor", "Fixed outdoor 1", "Fixed outdoor 2", "Fixed fluorescent 1", "Fixed fluorescent 2", "Hold current"]}, {["Auto", "Flicker-free 50 Hz", "Flicker-free 60 Hz", "Hold current"]}, {["None", "Prioritize frame rate", "Prioritize image quality"]}, {["Monochrome", "Color"]}] -> [_ _ _ _ _ w318]
          frame Default {
            w276 = FALSE ("Visible")
            w275 = FALSE ("Visible")
            n148 = property on="Motor" class="Clust (strict)"("Visible"=w275) -> ()  [unwired: 2 in, 2 out]
            n149 = property on="Test Ring" class="Ring (strict)"("Visible"=w275) -> ()  [unwired: 2 in, 2 out]
            n150 = property on="Rev/Fwd" class="Clust (strict)"("Visible"=w276) -> ()  [unwired: 2 in, 2 out]
            n151 = property on="On/Off" class="Bool (strict)"("Visible"=w276) -> ()  [unwired: 2 in, 2 out]
            n152 = property on="Test Slider" class="Slide (strict)"("Visible"=w276) -> ()  [unwired: 2 in, 2 out]
          }
          frame "Analog Out", "Motor", "PWM" {
            w282 = FALSE ("Visible")
            n153 = case shown="\"Analog Out\"" w281 {
              tunnel: [1.0 ("Value") -1.0 ("Value") 0.0 ("Value")] -> w280
              tunnel: [255.0 ("Value") 1.0 ("Value") 5.0 ("Value")] -> w279
              tunnel: [128.0 ("Value") 0.0 ("Value") 0.0 ("Value")] -> w278
              tunnel: [64.0 ("Value") 0.5 ("Value") 1.0 ("Value")] -> w277
              frame "PWM" {
              }
              frame "Motor", Default {
              }
              frame "Analog Out" {
              }
            }
            n154 = property on="Motor" class="Clust (strict)"("Visible"=TRUE) -> ()  [unwired: 2 in, 2 out]
            n155 = property on="Value" class="Slide (strict)"("Value"=w278, "Scale.Minimum"=w280, "Scale.Maximum"=w279, "Scale.Increment"=w277) -> ()  [unwired: 2 in, 2 out]
            n156 = property on="On/Off" class="Bool (strict)"("Visible"=w282) -> ()  [unwired: 2 in, 2 out]
            n157 = property on="Test Slider" class="Slide (strict)"("Visible"=w282) -> ()  [unwired: 2 in, 2 out]
            n158 = property on="Test Ring" class="Ring (strict)"("Visible"=w282) -> ()  [unwired: 2 in, 2 out]
            n159 = property on="Rev/Fwd" class="Clust (strict)"("Visible"=w282) -> ()  [unwired: 2 in, 2 out]
          }
          frame "Servo" {
            w298 = FALSE ("Visible")
            n160 = call <vilib>:"NT Read Number.vi"("Name"=w300) -> ("Numeric"=w299:dbl)  [unwired: 9 in, 1 out]
            n161 = property on="Test Slider" class="Slide (strict)"("Visible"=TRUE, "Scale.Maximum"=170.0 ("Scale.Range:Maximum")) -> ()  [unwired: 2 in, 2 out]
            n162 = local write "Test Slider"(w299) -> ()
            n163 = property on="Motor" class="Clust (strict)"("Visible"=w298) -> ()  [unwired: 2 in, 2 out]
            n164 = property on="Rev/Fwd" class="Clust (strict)"("Visible"=w298) -> ()  [unwired: 2 in, 2 out]
            n165 = property on="On/Off" class="Bool (strict)"("Visible"=w298) -> ()  [unwired: 2 in, 2 out]
            n166 = property on="Test Ring" class="Ring (strict)"("Visible"=w298) -> ()  [unwired: 2 in, 2 out]
          }
          frame "Relay", "Solenoid" {
            w301 = FALSE ("Visible")
            n167 = property on="Motor" class="Clust (strict)"("Visible"=w301) -> ()  [unwired: 2 in, 2 out]
            n168 = property on="Test Slider" class="Slide (strict)"("Visible"=w301) -> ()  [unwired: 2 in, 2 out]
            n169 = Search and Replace String(input string=w302, search string="/Value  **", replace string="/Direction") -> (result string=w308:string)  [unwired: 5 in, 3 out]
            n170 = property on="Test Ring" class="Ring (strict)"("Visible"=w301) -> ()  [unwired: 2 in, 2 out]
            n171 = call <vilib>:"NT Read String.vi"("Name"=w308) -> ("String"=w306:string)  [unwired: 9 in, 1 out]
            n172 = Equal?(x="Both directions", y=w306) -> (x = y?=w304:bool)
            n173 = Not(x=w304) -> (.not. x?=w305:bool)
            n174 = property on="Rev/Fwd" class="Clust (strict)"("Visible"=w304) -> ()  [unwired: 2 in, 2 out]
            n175 = property on="On/Off" class="Bool (strict)"("Visible"=w305, "Caption.Text"=w303) -> ()  [unwired: 2 in, 2 out]
          }
          frame "Compressor", "Digital Out" {
            w311 = FALSE ("Visible")
            # "Get direction and finish"
            n176 = property on="Motor" class="Clust (strict)"("Visible"=w311) -> ()  [unwired: 2 in, 2 out]
            n177 = property on="Test Slider" class="Slide (strict)"("Visible"=w311) -> ()  [unwired: 2 in, 2 out]
            n178 = property on="Test Ring" class="Ring (strict)"("Visible"=w311) -> ()  [unwired: 2 in, 2 out]
            n179 = property on="On/Off" class="Bool (strict)"("Visible"=TRUE, "Caption.Text"=w312) -> ()  [unwired: 2 in, 2 out]
            n180 = property on="Rev/Fwd" class="Clust (strict)"("Visible"=FALSE) -> ()  [unwired: 2 in, 2 out]
          }
          frame "Camera" {
            n181 = call <vilib>:"Get Last Path Segment.vi"("String in"=w319) -> ("String out"=w320:string)  [unwired: 10 in]
            n182 = property on="On/Off" class="Bool (strict)"("Visible"=FALSE) -> ()  [unwired: 2 in, 2 out]
            n183 = property on="Motor" class="Clust (strict)"("Visible"=FALSE) -> ()  [unwired: 2 in, 2 out]
            n184 = property on="Rev/Fwd" class="Clust (strict)"("Visible"=FALSE) -> ()  [unwired: 2 in, 2 out]
            n185 = case shown="\"White Balance  **\"" w320 {
              tunnel: w319 -> [w326 w335 w344 w353 w362 _ w368]
              tunnel: w318 -> [w324 w332 w341 w350 w359 _ _]
              frame "Size  **" {
                n186 = Index Array(array=w324) -> (element=w323:cluster{string[]})  [unwired: 1 in]
                n187 = call <vilib>:"NT Read String.vi"("Name"=w326) -> ("String"=w325:string)  [unwired: 9 in, 1 out]
                n188 = Unbundle(w323) -> (w321:string[])
                n189 = Match First String(2:w321, 3:w325) -> (0:w322:i32)  [unwired: 1 out]
                n190 = property on="Test Ring" class="Ring (strict)"("Value"=w322, "Strings []"=w321) -> ()  [unwired: 2 in, 2 out]
                n191 = property on="Test Ring" class="Ring (strict)"("Visible"=TRUE) -> ()  [unwired: 2 in, 2 out]
                n192 = property on="Test Slider" class="Slide (strict)"("Visible"=FALSE) -> ()  [unwired: 2 in, 2 out]
              }
              frame "White Balance  **" {
                n193 = Index Array(array=w332, index=1) -> (element=w333:cluster{string[]})
                n194 = call <vilib>:"NT Read String.vi"("Name"=w335) -> ("String"=w334:string)  [unwired: 9 in, 1 out]
                n195 = Unbundle(w333) -> (w330:string[])
                n196 = Match First String(2:w330, 3:w334) -> (0:w329:i32)  [unwired: 1 out]
                n197 = property on="Test Ring" class="Ring (strict)"("Value"=w329, "Strings []"=w330) -> ()  [unwired: 2 in, 2 out]
                n198 = property on="Test Ring" class="Ring (strict)"("Visible"=TRUE) -> ()  [unwired: 2 in, 2 out]
                n199 = property on="Test Slider" class="Slide (strict)"("Visible"=FALSE) -> ()  [unwired: 2 in, 2 out]
              }
              frame "Exposure  **" {
                n200 = Index Array(array=w341, index=2) -> (element=w342:cluster{string[]})
                n201 = call <vilib>:"NT Read String.vi"("Name"=w344) -> ("String"=w343:string)  [unwired: 9 in, 1 out]
                n202 = Unbundle(w342) -> (w338:string[])
                n203 = Match First String(2:w338, 3:w343) -> (0:w339:i32)  [unwired: 1 out]
                n204 = property on="Test Ring" class="Ring (strict)"("Value"=w339, "Strings []"=w338) -> ()  [unwired: 2 in, 2 out]
                n205 = property on="Test Ring" class="Ring (strict)"("Visible"=TRUE) -> ()  [unwired: 2 in, 2 out]
                n206 = property on="Test Slider" class="Slide (strict)"("Visible"=FALSE) -> ()  [unwired: 2 in, 2 out]
              }
              frame "Exposure Priority  **" {
                n207 = Index Array(array=w350, index=3) -> (element=w351:cluster{string[]})
                n208 = call <vilib>:"NT Read String.vi"("Name"=w353) -> ("String"=w352:string)  [unwired: 9 in, 1 out]
                n209 = Unbundle(w351) -> (w347:string[])
                n210 = Match First String(2:w347, 3:w352) -> (0:w348:i32)  [unwired: 1 out]
                n211 = property on="Test Ring" class="Ring (strict)"("Value"=w348, "Strings []"=w347) -> ()  [unwired: 2 in, 2 out]
                n212 = property on="Test Ring" class="Ring (strict)"("Visible"=TRUE) -> ()  [unwired: 2 in, 2 out]
                n213 = property on="Test Slider" class="Slide (strict)"("Visible"=FALSE) -> ()  [unwired: 2 in, 2 out]
              }
              frame "Color Enable  **" {
                n214 = Index Array(array=w359, index=4) -> (element=w360:cluster{string[]})
                n215 = call <vilib>:"NT Read String.vi"("Name"=w362) -> ("String"=w361:string)  [unwired: 9 in, 1 out]
                n216 = Unbundle(w360) -> (w356:string[])
                n217 = Match First String(2:w356, 3:w361) -> (0:w357:i32)  [unwired: 1 out]
                n218 = property on="Test Ring" class="Ring (strict)"("Value"=w357, "Strings []"=w356) -> ()  [unwired: 2 in, 2 out]
                n219 = property on="Test Ring" class="Ring (strict)"("Visible"=TRUE) -> ()  [unwired: 2 in, 2 out]
                n220 = property on="Test Slider" class="Slide (strict)"("Visible"=FALSE) -> ()  [unwired: 2 in, 2 out]
              }
              frame Default {
                n221 = property on="Test Ring" class="Ring (strict)"("Visible"=FALSE) -> ()  [unwired: 2 in, 2 out]
                n222 = property on="Test Slider" class="Slide (strict)"("Visible"=FALSE) -> ()  [unwired: 2 in, 2 out]
              }
              frame "Brightness  **", "Color Level  **", "Compression  **", "FPS  **", "Sharpness  **" {
                n223 = call <vilib>:"NT Read Number.vi"("Name"=w368) -> ("Numeric"=w367:dbl)  [unwired: 9 in, 1 out]
                n224 = local write "Test Slider"(w367) -> ()
                n225 = property on="Test Slider" class="Slide (strict)"("Visible"=TRUE, "Scale.Maximum"=100.0 ("Scale.Range:Maximum")) -> ()  [unwired: 2 in, 2 out]
                n226 = property on="Test Ring" class="Ring (strict)"("Visible"=FALSE) -> ()  [unwired: 2 in, 2 out]
              }
            }
          }
        }
        n227 = property on="Progress" class="Clust (strict)"("Visible"=FALSE) -> ()  [unwired: 2 in, 2 out]
      }
      event "Test Name": Mouse Enter {
        # "Populate the ring with the list of tests"
        n228 = event-data() -> ()  [unwired: 1 in, 1 out]
        n229 = call <vilib>:"NT Read String Array.vi"("Name"="TestMode/TestList") -> ("String Array"=w376:string[])  [unwired: 9 in, 1 out]
        n230 = Build Array (concatenate)("Select the test to run...", w376) -> (w375:string[])
        n231 = property on="Test Name" class="Ring (strict)"("Strings []"=w375) -> ()  [unwired: 2 in, 2 out]
      }
      event "Test Name": Value Change {
        w378 = FALSE ("Visible")
        # "Tell the robot the test name to run"
        n232 = event-data() -> ("NewVal"=w382:u16)  [unwired: 1 in]
        n233 = property on="Test Name" class="Ring (strict)"() -> ("Strings []"=w383:string[])  [unwired: 2 in, 2 out]
        n234 = local write "Progress"(T6 {"Test Progress"=0, "Test Progress Text"=""} ("Progress")) -> ()
        n235 = Index Array(array=w383, index=w382) -> (element=w381:string)
        n236 = call <vilib>:"NT Write String.vi"("String"=w381, "Name"="TestMode/TestName") -> ()  [unwired: 9 in, 1 out]
        n237 = property on="Progress" class="Clust (strict)"("Visible"=TRUE) -> ()  [unwired: 2 in, 2 out]
        n238 = property on="Motor" class="Clust (strict)"("Visible"=w378) -> ()  [unwired: 2 in, 2 out]
        n239 = property on="Test Slider" class="Slide (strict)"("Visible"=w378) -> ()  [unwired: 2 in, 2 out]
        n240 = property on="On/Off" class="Bool (strict)"("Visible"=w378) -> ()  [unwired: 2 in, 2 out]
        n241 = property on="Rev/Fwd" class="Clust (strict)"("Visible"=w378) -> ()  [unwired: 2 in, 2 out]
        n242 = property on="Test Ring" class="Ring (strict)"("Visible"=w378) -> ()  [unwired: 2 in, 2 out]
      }
      event "Select Auto": Mouse Enter {
        # "Populate the combo box with the list of autonomous options"
        n243 = event-data() -> ()  [unwired: 1 in, 1 out]
        n244 = call <vilib>:"NT Read String Array.vi"("Name"="Auto List") -> ("String Array"=w385:string[])  [unwired: 9 in, 1 out]
        n245 = property on="Select Auto" class="CmbBox"("Strings[]"=w385) -> ()  [unwired: 2 in, 2 out]
      }
      event "Select Auto": Value Change {
        # "User modified the Auto Selection. Write to NT variable so robot knows."
        n246 = event-data() -> ("NewVal"=w388:string)  [unwired: 1 in]
        n247 = call <vilib>:"NT Write String.vi"("String"=w388, "Name"="Auto Selector") -> ()  [unwired: 9 in, 1 out]
      }
      event "Command Selection": Value Change {
        # "Get the params and show in table"
        n248 = event-data() -> ("NewVal"=w394:i32)  [unwired: 1 in]
        n249 = property on="Command Selection" class="MCListbox (strict)"() -> ("ItemNames"=w392:string[][])  [unwired: 2 in, 2 out]
        n250 = call <vilib>:"WPI_DashboardUpdate Command Params.vi"("NewVal"=w394, "Commands"=w392, "Param Tbl"=w393) -> ()  [unwired: 8 in, 1 out]
      }
      event "Execute Command": Value Change {
        # "Started one, Unique ID holds\nresponse"
        n251 = event-data() -> ()  [unwired: 1 in, 1 out]
        n252 = property on="Command Selection" class="MCListbox (strict)"() -> ("ItemNames"=w405:string[][])  [unwired: 2 in, 2 out]
        n253 = Index Array(array=w405, index (row)="Command Selection", index (col)=0) -> (element=w403:string)
        n254 = call <vilib>:"Invoke Commands.vi"("Command Params"="Command Params", "Function Name"=w403) -> ("Params"=w399:u8, "Started"=w398:bool)  [unwired: 7 in, 1 out]
        n255 = Array Subset(array="Command Params", length (row)=w399) -> (w400:string[][])  [unwired: 3 in]
        n256 = Select(t="Executing" ("Cmd Status"), s=w398, f="" ("Cmd Status")) -> (s? t:f=→"Cmd Status":string)
      }
      event "Command Selection": Double Click {
        n257 = event-data() -> ("Row"=w413:i32)  [unwired: 1 in]
        n258 = property on="Command Selection" class="MCListbox (strict)"() -> ("ItemNames"=w416:string[][])  [unwired: 2 in, 2 out]
        n259 = local read "Command Params"() -> (w412:string[][])
        n260 = Index Array(array=w416, index (row)=w413, index (col)=0) -> (element=w414:string)
        n261 = call <vilib>:"Invoke Commands.vi"("Command Params"=w412, "Function Name"=w414) -> ("Params"=w411:u8, "Started"=w406:bool)  [unwired: 7 in, 1 out]
        n262 = Array Subset(array=w412, length (row)=w411) -> (w410:string[][])  [unwired: 3 in]
        n263 = Select(t="Executing" ("Cmd Status"), s=w406, f="" ("Cmd Status")) -> (s? t:f=w407:string)
        n264 = local write "Cmd Status"(w407) -> ()
      }
      event "CheckList": Double Click {
        # "Shift clears all"
        # "Update symbols on the listbox"
        n265 = event-data() -> ("PlatMods.Shift"=w418:bool, "Row"=w420:i32)  [unwired: 1 in]
        n266 = case shown="True" w418 {
          tunnel: w420 -> [w424 _]
          tunnel: 1 -> [w423 _]
          frame False {
            n267 = property on="CheckList" class="LstBox (strict)"() -> ("Item Symbols"=w422:i32[])  [unwired: 2 in, 2 out]
            n268 = Replace Array Subset(array=w422, new element=w423, index=w424) -> (w421:i32[])
            n269 = property on="CheckList" class="LstBox (strict)"("Item Symbols"=w421) -> ()  [unwired: 2 in, 2 out]
          }
          frame True {
            w425 = 0 ("Top Row")
            n270 = property on="CheckList" class="LstBox (strict)"() -> ("Number of Rows"=w427:u32)  [unwired: 2 in, 2 out]
            n271 = Initialize Array(0, w427) -> (w426:i32[])
            n272 = property on="CheckList" class="LstBox (strict)"("Top Row"=w425, "Value"=w425, "Item Symbols"=w426) -> ()  [unwired: 2 in, 2 out]
          }
        }
      }
      event "CheckList": Key Down {
        # "Update symbols on the listbox\nLeft and right keys check and uncheck"
        n273 = event-data() -> ("VKey"=w431:T22)  [unwired: 1 in]
        n274 = case shown="\"Left\", \"Right\"" w431 {
          selector: w431 -> [w436 _]
          tunnel: eventvkey."Left" ("VKey") -> [w434 _]
          frame "Left", "Right" {
            n275 = Equal?(x=w434, y=w436) -> (x = y?=w435:bool)
            n276 = Select(t=0, s=w435, f=1) -> (s? t:f=w437:i32)
            n277 = property on="CheckList" class="LstBox (strict)"() -> ("Item Symbols"=w440:i32[])  [unwired: 2 in, 2 out]
            n278 = Replace Array Subset(array=w440, new element=w437, index="CheckList") -> (w439:i32[])
            n279 = property on="CheckList" class="LstBox (strict)"("Item Symbols"=w439) -> ()  [unwired: 2 in, 2 out]
          }
          frame Default {
          }
        }
      }
      event "Motor.Enable": Value Change {
        # "When the test mode otor enable helper is set, update that\ntree row item's value"
        n280 = event-data() -> ("NewVal"=w446:bool)  [unwired: 1 in]
        n281 = Unbundle("Motor") -> ("Value"=w445:dbl)  [unwired: 1 out]
        n282 = Select(t=w445, s=w446, f=0.0) -> (s? t:f=w443:dbl)
        n283 = call <vilib>:"NT Write Number.vi"("Numeric"=w443, "Name"=w442) -> ()  [unwired: 9 in, 1 out]
      }
      event "Test Slider": Value Change {
        # "When the test mode slider helper is set, update that\ntree row item's value"
        n284 = event-data() -> ("NewVal"=w449:dbl)  [unwired: 1 in]
        n285 = call <vilib>:"NT Write Number.vi"("Numeric"=w449, "Name"=w450) -> ()  [unwired: 9 in, 1 out]
      }
      event "On/Off": Value Change {
        # "When the test mode on/off helper value is set, update that\ntree row item's value"
        n286 = event-data() -> ("NewVal"=w454:bool)  [unwired: 1 in]
        n287 = Boolean To (0,1)(Boolean=w454) -> (0, 1=w453:i16)
        n288 = call <vilib>:"NT Write Number.vi"("Numeric"=w453, "Name"=w452) -> ()  [unwired: 9 in, 1 out]
      }
      event "Rev/Fwd": Value Change {
        # "When the test mode helper value for relays is set, update that\ntree row item's value"
        n289 = event-data() -> ("NewVal.Forward"=w462:bool, "NewVal.Reverse"=w461:bool)  [unwired: 1 in]
        n290 = Boolean To (0,1)(Boolean=w462) -> (0, 1=w458:i16)
        n291 = Boolean To (0,1)(Boolean=w461) -> (0, 1=w460:i16)
        n292 = Negate(x=w460) -> (-x=w459:i16)
        n293 = Add(x=w458, y=w459) -> (x+y=w457:i16)
        n294 = call <vilib>:"NT Write Number.vi"("Numeric"=w457, "Name"=w456) -> ()  [unwired: 9 in, 1 out]
      }
      event "Test Ring": Value Change {
        # "When a test mode helper value is selected from the ring,\nset the tree item's variable to the string value"
        n295 = event-data() -> ("NewVal"=w466:u16)  [unwired: 1 in]
        n296 = property on="Test Ring" class="Ring (strict)"() -> ("Strings []"=w467:string[])  [unwired: 2 in, 2 out]
        n297 = Index Array(array=w467, index=w466) -> (element=w465:string)
        n298 = call <vilib>:"NT Write String.vi"("String"=w465, "Name"=w464) -> ()  [unwired: 9 in, 1 out]
      }
      event "Rec Mode": Value Change {
        # "Update globals for recording mode and path to read log from.\nClear when logging and let NetworkTables set path for vision to\nuse."
        n299 = event-data() -> ("NewVal"=w478:enum32{"Stop", "Record", "Playback"})  [unwired: 1 in]
        n300 = global write "WPI_DashboardLogging Global.vi" "Logging Filename"(path "") -> ()
        n301 = global write "WPI_DashboardLogging Global.vi" "Recording"(w478) -> ()
        n302 = case shown="\"Playback\"" w478 {
          tunnel: w477 -> [_ w480 w489]
          tunnel: [_ _ w488] -> w475
          tunnel: [_ _ w487] -> _
          tunnel: w473 -> [_ _ w485]
          tunnel: cluster{i32, i32} {-250, 170} -> [_ _ w484]
          tunnel: [_ _ T23 {"Image Size"=TRUE, "Image Type"=TRUE, "Pixel Value"=TRUE, "ROI Information"=TRUE, "Zoom Factor"=FALSE} ("Image Information Shown:All Elements")] -> w468
          tunnel: [_ _ TRUE ("Zoom Factor")] -> w469
          tunnel: w471 -> [_ _ w481]
          frame Default {
          }
          frame "Stop", "Record" {
            # "Place Window too"
            n303 = invoke class="VI" method="FP.Close"(reference=w480) -> (reference out=w479:refnum<vi>)  [unwired: 2 in, 2 out]
            n304 = invoke class="VI" method="Abort VI"(reference=w479) -> ()  [unwired: 2 in, 3 out]
          }
          frame "Playback" {
            n305 = call "Open Playback Panel.vi"("Offset"=w484, "DB VI Ref"=w485, "Playback in"=w489) -> ("Playback out"=w486:refnum<vi>)  [unwired: 8 in]
            n306 = register-events(w486, w481) -> (reference out=w488:refnum<event-registration>, error out=w487:errorcluster)  [unwired: 2 in]
          }
        }
        n307 = property on="Camera Image Right" class="ImageControl"("Image Information Shown"=w468, "Image Information Visible"=w469) -> ()  [unwired: 2 in, 2 out]
        n308 = property on="Camera Image" class="ImageControl"("Image Information Shown"=w468, "Image Information Visible"=w469) -> ()  [unwired: 2 in, 2 out]
        n309 = call <vilib>:"WPI_DashboardNT Log FieldName Cache.vi"("Operation"=enum16{"Lookup/Add", "Index", "Clear"}."Clear") -> ()  [unwired: 8 in, 3 out]
      }
      event Panel Close {
        w491 = enum32{"Stop", "Record", "Playback"}."Stop" ("Rec Mode")
        # "Playback window has been closed, abort"
        n310 = event-data() -> ()  [unwired: 1 in, 4 out]
        n311 = local write "Rec Mode"(w491) -> ()
        n312 = global write "WPI_DashboardLogging Global.vi" "Recording"(w491) -> ()
      }
      event Panel Close {
        # "Abort playback window and ourself"
        n313 = event-data() -> ()  [unwired: 1 in, 4 out]
        n314 = invoke class="VI" method="FP.Close"(reference=w495) -> (reference out=w494:refnum<vi>)  [unwired: 2 in, 2 out]
        n315 = invoke class="VI" method="Abort VI"(reference=w494) -> (error out=w493:errorcluster)  [unwired: 2 in, 2 out]
        n316 = invoke class="VI" method="Abort VI"(error in=w493) -> ()  [unwired: 2 in, 3 out]
      }
      event User Event {
        n317 = event-data() -> ("IDs"=w502:cluster{"RPC field ID":u16, "Unique ID":u16}, "String"=w501:string)  [unwired: 1 in]
        n318 = Bundle("IDs"=w502, "String"=w501) -> (w500:T9)  [unwired: 1 in]
        n319 = call <vilib>:"Retrieve RPC Response.vi"("RPC Response"=w500) -> ("Output"=w498:string[][])  [unwired: 10 in]
        n320 = Build Array (concatenate)(w496, w498) -> (w497:string[][])
        n321 = local write "Command Params"(w497) -> ()
        n322 = local write "Cmd Status"("" ("Cmd Status")) -> ()
      }
      event "Tree": Double Click {
        n323 = event-data() -> ("PlatMods"=w508:T26, "Tag"=w505:string)  [unwired: 1 in]
        n324 = Unbundle(w508) -> ("Shift"=w507:bool)  [unwired: 4 out]
        n325 = String Subset(string=w505, length (rest)=1 ("length (rest)")) -> (substring=w504:string)  [unwired: 1 in]
        n326 = Not(x=w507) -> (.not. x?=w506:bool)
        n327 = case shown="\"/\"" w504 {
          tunnel: w505 -> [_ w511]
          tunnel: w506 -> [_ w510]
          frame Default {
          }
          frame "/" {
            n328 = call <vilib>:"NT Update Persistence.vi"("Persistence"=w510, "Name"=w511) -> ()  [unwired: 9 in, 1 out]
          }
        }
      }
    }
  }
  n329 = local write "Dashboard Tab"(T2."Drive" ("Dashboard Tab")) -> ()
  n330 = property on="On/Off" class="Bool (strict)"("Visible"=w36) -> ()  [unwired: 2 in, 2 out]
  n331 = property on="Motor" class="Clust (strict)"("Visible"=w36) -> ()  [unwired: 2 in, 2 out]
  n332 = property on="Progress" class="Clust (strict)"("Visible"=w36) -> ()  [unwired: 2 in, 2 out]
  n333 = property on="Test Ring" class="Ring (strict)"("Visible"=w36) -> ()  [unwired: 2 in, 2 out]
  n334 = property on="Rev/Fwd" class="Clust (strict)"("Visible"=w36) -> ()  [unwired: 2 in, 2 out]
  n335 = while {
    tunnel: u16 1741 ("timeout ms (25000)") -> [w513]
    stop <- FALSE stop-if-true
    n336 = TCP Create Listener(10:w513) -> (0:w512:errorcluster, 3:w514:refnum<k5>)  [unwired: 4 in, 1 out]
    n337 = case shown="No Error" w512 {
      selector: w512 -> [w516 _]
      tunnel: w514 -> [w517 _]
      frame No Error {
        n338 = while {
          tunnel: w517 -> [w520]
          tunnel: w516 -> [w519]
          stop <- FALSE stop-if-true
          n339 = TCP Wait On Listener(8:w519, 11:w520) -> (0:w521:errorcluster, 4:w522:refnum<k5>)  [unwired: 2 in, 3 out]
          n340 = local write "TCP"(w522) -> ()
          n341 = case shown="No Error" w521 {
            frame No Error {
            }
            frame Error {
              n342 = Wait (ms)(milliseconds to wait=u32 1000) -> ()  [unwired: 1 out]
            }
          }
        }
      }
      frame Error {
        n343 = Wait (ms)(milliseconds to wait=u32 1000) -> ()  [unwired: 1 out]
      }
    }
  }
  n344 = local write "Command Selection"(u16 0 ("milliseconds to wait")) -> ()
  n345 = local write "Command Params"(string[][] [] ("Command Params")) -> ()
  n346 = global write "WPI_DashboardLogging Global.vi" "Recording"(w59) -> ()
  n347 = local write "Rec Mode"(w59) -> ()
  n348 = call <vilib>:"NT Write String.vi"("String"="Select Auto", "Name"="Auto Selector") -> ()  [unwired: 9 in, 1 out]
